vi "Auto Loop 0.vi"(10 "auto #":u32, 11 "Call Context":T1) -> (0 "Loop 0 Value2":dbl, 1 "Loop 0 Value1":dbl, 2 "Loop 0 exit value":i32, 3 "Loop 0 SubState":T2=enum."auto")   [LabVIEW 2011]
uses:
  subStates.ctl
  <vilib>/Rock Robotics/WPI/DriverStation/WPI_DriverStationDerivedRobotMode.ctl
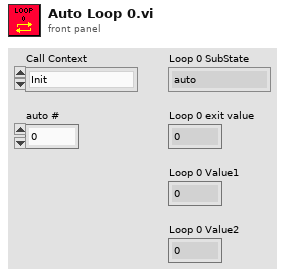
[diagram p1: front panel]
types:
  T1 = typedef "WPI_DriverStationDerivedRobotMode.ctl" = enum16{"Init", "Execute", "Stop"}
  T2 = typedef "subStates.ctl" = enum16{"null", "wait", "driver control", "auto", "manual override", "autoDrive", "hold position", "rotate", "end"}
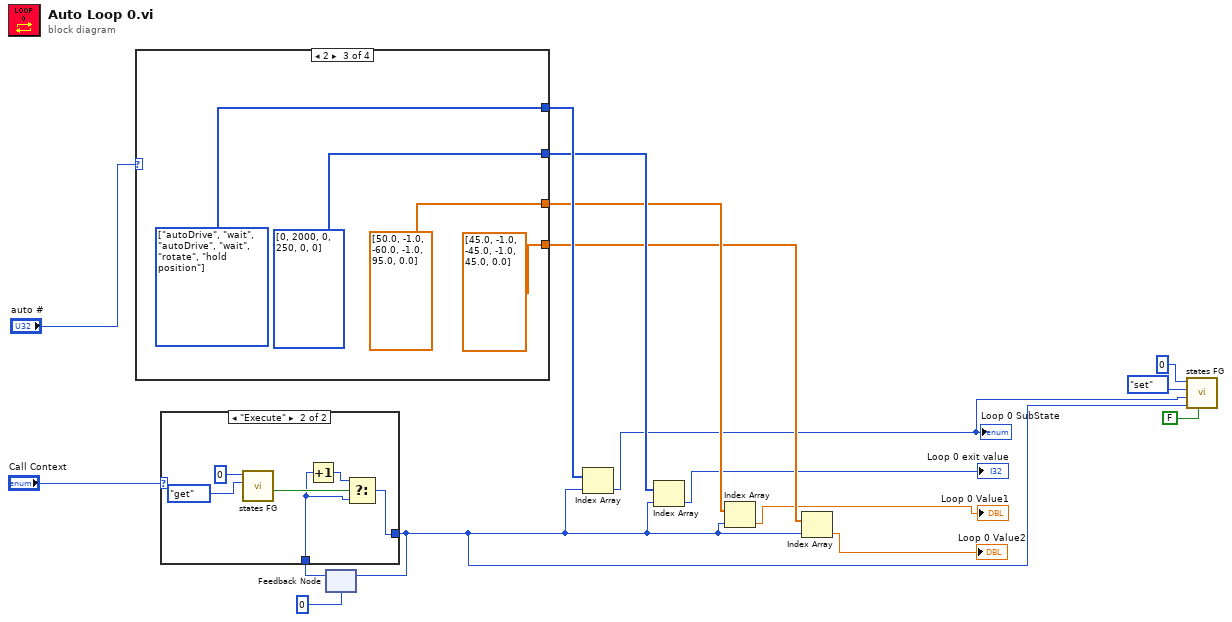
[diagram p0: block diagram]
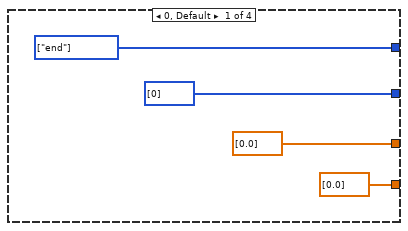
[diagram p2: hidden frame]
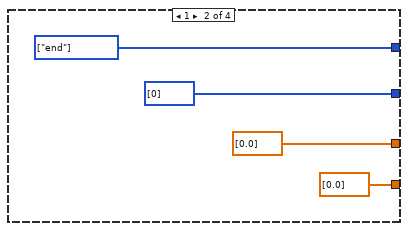
[diagram p3: hidden frame]
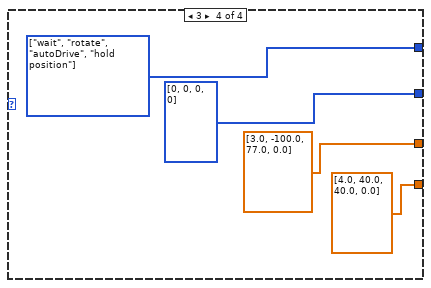
[diagram p4: hidden frame]
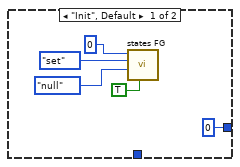
[diagram p5: hidden frame]
diagram:
  n1 = case shown="2" "auto #" {
    tunnel: [dbl[] [0.0] ("value2 array") dbl[] [0.0] ("value2 array") dbl[] [45.0, -1.0, -45.0, -1.0, 45.0, 0.0] ("value2 array") dbl[] [4.0, 40.0, 40.0, 0.0] ("value2 array")] -> w8
    tunnel: [dbl[] [0.0] ("value1 array") dbl[] [0.0] ("value1 array") dbl[] [50.0, -1.0, -60.0, -1.0, 95.0, 0.0] ("value1 array") dbl[] [3.0, -100.0, 77.0, 0.0] ("value1 array")] -> w9
    tunnel: [w18 w22 w26 w30] -> w11
    tunnel: [i32[] [0] ("exit value array") i32[] [0] ("exit value array") i32[] [0, 2000, 0, 250, 0, 0] ("exit value array") i32[] [0, 0, 0, 0] ("exit value array")] -> w10
    frame 0, Default {
      w18 = T2[] [enum."end"] items=["null", "wait", "driver control", "auto", "manual override", "autoDrive", "hold position", "rotate", "end"] ("substate array")
    }
    frame 1 {
      w22 = T2[] [enum."end"] items=["null", "wait", "driver control", "auto", "manual override", "autoDrive", "hold position", "rotate", "end"] ("substate array")
    }
    frame 2 {
      w26 = T2[] [enum."autoDrive", enum."wait", enum."autoDrive", enum."wait", enum."rotate", enum."hold position"] items=["null", "wait", "driver control", "auto", "manual override", "autoDrive", "hold position", "rotate", "end"] ("substate array")
    }
    frame 3 {
      w30 = T2[] [enum."wait", enum."rotate", enum."autoDrive", enum."hold position"] items=["null", "wait", "driver control", "auto", "manual override", "autoDrive", "hold position", "rotate", "end"] ("substate array")
    }
  }
  n2 = feedback #1(0 ("Value1 2")) -> (w13:i32)
  n3 = case shown="\"Execute\"" "Call Context" {
    tunnel: [0 ("Value1 2") w42] -> w2
    tunnel: w13 -> [_ w39]
    frame "Init", Default {
      n4 = call "states FG.vi"("exit in"=TRUE, "subState in"=subStates."null", "menu (get)"=enum16{"set", "get"}."set", "Loop ID"=0) -> ()  [unwired: 4 in, 4 out]
    }
    frame "Execute" {
      n5 = call "states FG.vi"("menu (get)"=enum16{"set", "get"}."get", "Loop ID"=0) -> ("exit out"=w41:bool)  [unwired: 6 in, 3 out]
      n6 = Increment(x=w39) -> (x+1=w43:i32)
      n7 = Select(t=w43, s=w41, f=w39) -> (s? t:f=w42:i32)
    }
  }
  n8 = feedback-in #1(w2) -> ()
  n9 = Index Array(array=w11, index=w2) -> (element=w1:T2)
  "Loop 0 SubState" <- w1
  n10 = Index Array(array=w10, index=w2) -> (element=→"Loop 0 exit value":i32)
  n11 = Index Array(array=w9, index=w2) -> (element=→"Loop 0 Value1":dbl)
  n12 = Index Array(array=w8, index=w2) -> (element=→"Loop 0 Value2":dbl)
  n13 = call "states FG.vi"("exit in"=FALSE, "state # in"=w2, "subState in"=w1, "menu (get)"=enum16{"set", "get"}."set", "Loop ID"=0) -> ()  [unwired: 3 in, 4 out]
